vi "Get Discovery Service Address.vi"(8 "error in":errorcluster, 11 "cluster id (\"\")":string) -> (0 "error out":errorcluster, 3 "address":string)   [LabVIEW 2020, in "MeasurementTemplate_server.lvlib"]
uses:
  MeasurementTemplate_server.lvlib
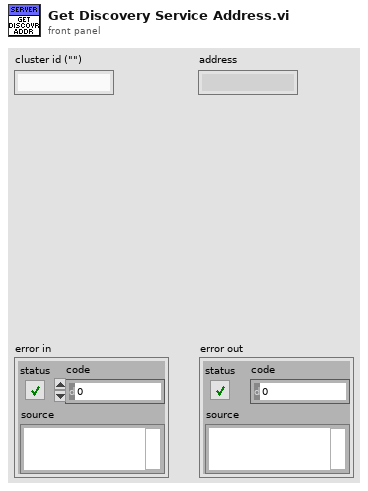
[diagram p1: front panel]
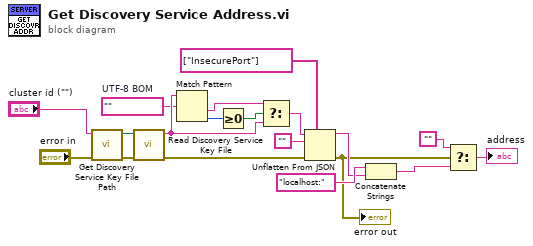
[diagram p0: block diagram]
diagram:
  w9 = "﻿"  # UTF-8 BOM
  n1 = call "Get Discovery Service Key File Path.vi"("error in (no error)"="error in", "cluster id (\"\")"="cluster id (\"\")") -> ("error out"=w16:errorcluster, "key file path"=w17:path)  [unwired: 8 in]
  n2 = call "Read Discovery Service Key File.vi"("error in (no error)"=w16, "key file path"=w17) -> ("error out"=w7:errorcluster, "key json"=w10:string)  [unwired: 8 in]
  n3 = Match Pattern(string=w10, regular expression=w9) -> (after substring=w13:string, offset past match=w12:i32)  [unwired: 1 in, 2 out]
  n4 = Greater Or Equal To 0?(x=w12) -> (x >= 0?=w14:bool)
  n5 = Select(t=w13, s=w14, f=w10) -> (s? t:f=w15:string)
  n6 = Unflatten From JSON(path=string[] ["InsecurePort"], JSON string=w15, type and defaults="", error in (no error)=w7) -> (value=w5:string, error out=w4:errorcluster)  [unwired: 3 in]
  "error out" <- w4
  n7 = Concatenate Strings("localhost:", w5) -> (w2:string)
  n8 = Select(t="", s=w4, f=w2) -> (s? t:f=→"address":string)
